vi "Insert Data by String Array.vi"(7 "data":string[](array[string]), 8 "error in (no error)":errorcluster, 9 "columns":string[](array[string]), 10 "table":string, 11 "Database Interface in":refnum<class "Database Interface.lvclass">) -> (0 "error out":errorcluster, 3 "Database Interface out":refnum<class "Database Interface.lvclass">)   [LabVIEW 2020, in "Database Interfaces.lvlib" / "Database Interface.lvclass"]
uses:
  Database Interface.lvclass
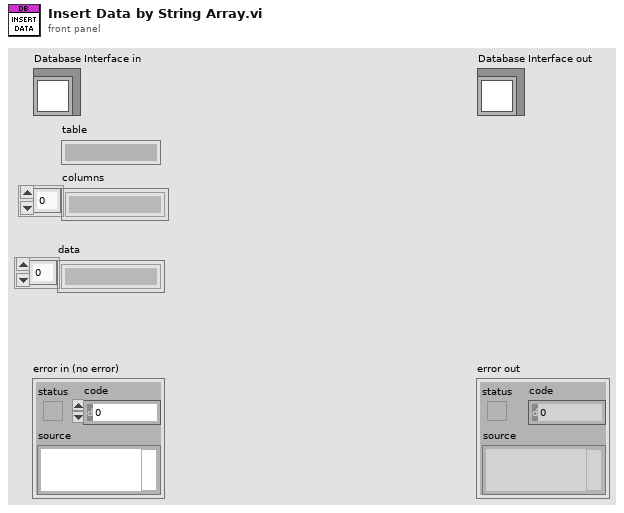
[diagram p1: front panel]
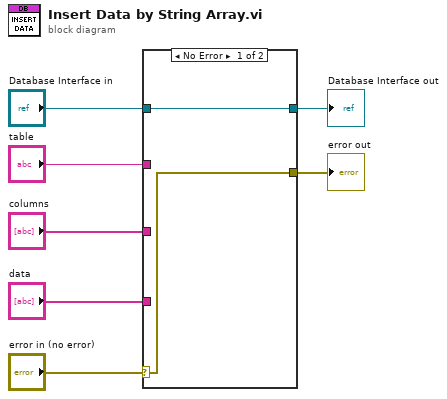
[diagram p0: block diagram]
diagram:
  n1 = case shown="No Error" "error in (no error)" {
    selector: "error in (no error)" -> [w9 w11]
    tunnel: [w9 w11] -> w6
    tunnel: [w8 w10] -> w4
    tunnel: "Database Interface in" -> [w8 w10]
    tunnel: "table" -> [_ _]
    tunnel: "columns" -> [_ _]
    tunnel: "data" -> [_ _]
    frame No Error {
    }
    frame Error {
    }
  }
  "error out" <- w6
  "Database Interface out" <- w4
